vi "Start.vi"(8 "error in (no error)":errorcluster, 11 "1553 Board in":refnum<class "1553 Session.lvclass">) -> (0 "error out":errorcluster, 3 "1553 Board out":refnum<class "1553 Session.lvclass">)   [LabVIEW 2020, in "BCI-1553 API.lvlib" / "1553 Session.lvclass"]
doc: "Starts a configured 1553 Session."
uses:
  1553 Session.lvclass
  1553 Session.lvclass/1553 Session.ctl
  1553 Component/1553 Component.lvclass
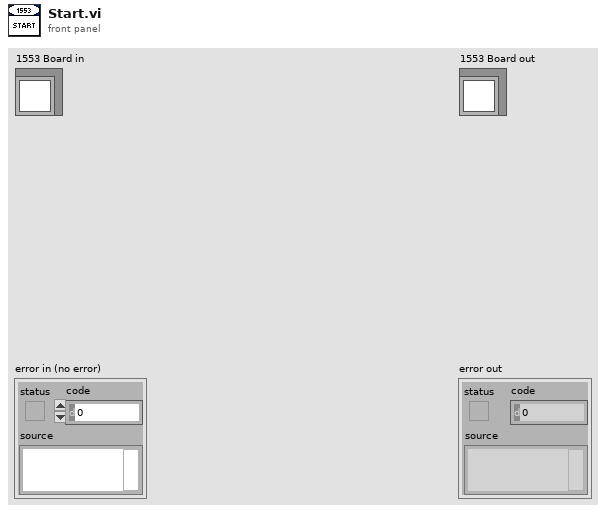
[diagram p1: front panel]
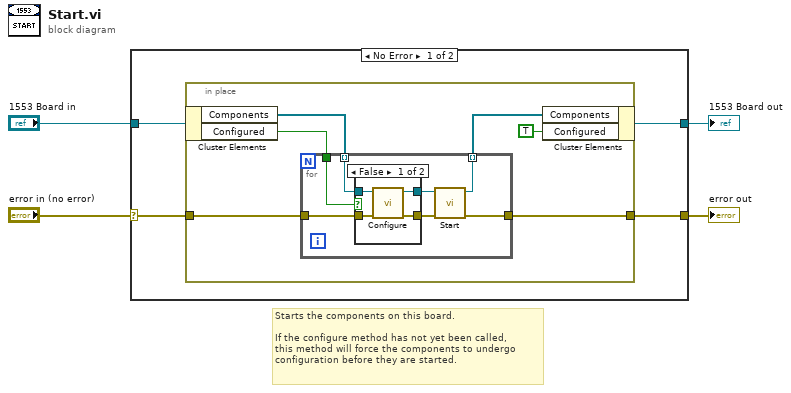
[diagram p0: block diagram]
diagram:
  # "Starts the components on this board.\n\nIf the configure method has not yet been called,\nthis method will force the components to undergo\nconfiguration before they are started."
  n1 = case shown="No Error" "error in (no error)" {
    selector: "error in (no error)" -> [w7 w29]
    tunnel: [w6 w29] -> w3
    tunnel: [w5 w28] -> w1
    tunnel: "1553 Board in" -> [w8 w28]
    frame No Error {
      n2 = in-place {
        in-place-border: w7 -> [w14]
        in-place-border: [w11] -> w6
        n3 = in-place-cluster #1(w8) -> ("Components"=w13:refnum<class "1553 Component.lvclass">[], "Configured"=w10:bool)
        n4 = for {
          tunnel: w14 -> [w17]
          tunnel: [w21] -> w11
          tunnel: w13 -> [w19] mode=indexing
          tunnel: [w20] -> w12 mode=indexing
          tunnel: w10 -> [w15]
          n5 = case shown="False" w15 {
            tunnel: w19 -> [w25 w27]
            tunnel: [w24 w27] -> w18
            tunnel: w17 -> [w23 w26]
            tunnel: [w22 w26] -> w16
            frame False {
              n6 = call-dynamic "Configure.vi"("error in (no error)"=w23, "1553 Component in"=w25) -> ("error out"=w22:errorcluster, "1553 Component out"=w24:refnum<class "1553 Component.lvclass">)  [unwired: 8 in]
            }
            frame True {
            }
          }
          n7 = call-dynamic "Start.vi"("error in (no error)"=w16, "1553 Component in"=w18) -> ("error out"=w21:errorcluster, "1553 Component out"=w20:refnum<class "1553 Component.lvclass">)  [unwired: 8 in]
        }
        n8 = in-place-cluster #1("Components"=w12, "Configured"=TRUE) -> (w5:refnum<class "1553 Session.lvclass">)
      }
    }
    frame Error {
    }
  }
  "error out" <- w3
  "1553 Board out" <- w1
